vi "Rename State in Schedule.vi"(0 "Tosca in":refnum<class "Parameters.lvclass">, 5 "Old Name":string, 7 "New Name":string, 11 "error in (no error)":errorcluster) -> (4 "Tosca out":refnum<class "Parameters.lvclass">, 15 "error out":errorcluster)   [LabVIEW 2015, in "Parameters.lvclass"]
uses:
  Parameters.lvclass
  Parameters.lvclass/Parameters.ctl
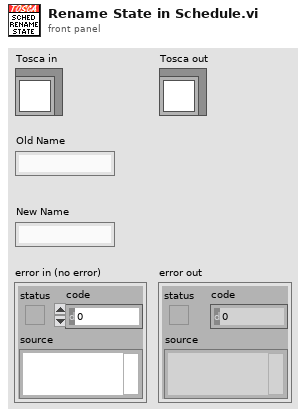
[diagram p1: front panel]
types:
  T1 = typedef "Tosca-Parameter Family.ctl" = cluster{"Name":string, "Number":i32, "Vars":T2[], "Mask":bool[][], "one each":bool}
  T2 = typedef "Tosca-Parameter Table Element.ctl" = cluster{"state":string, "chan":string, "param":string, "expr":string, "dim":T3, "value":dbl[]}
  T3 = typedef "Tosca-Parameter Dimension.ctl" = enum16{"Ind", "X", "Y"}
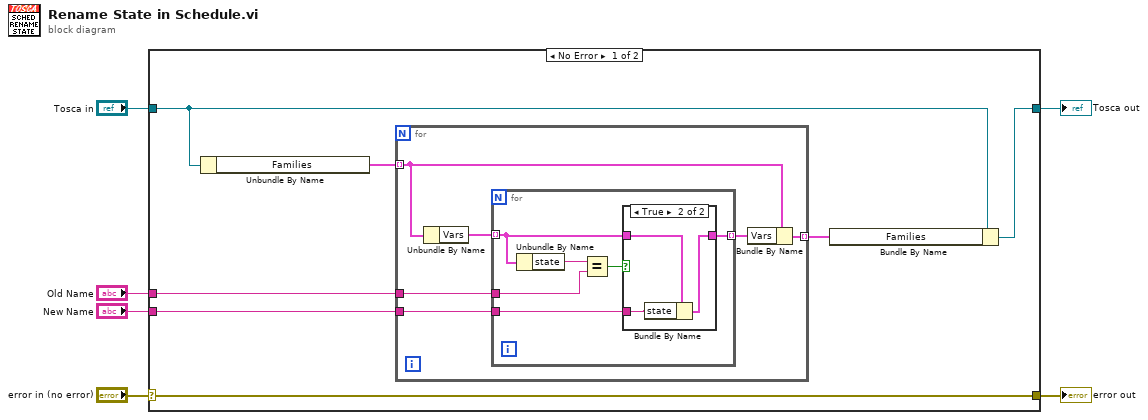
[diagram p0: block diagram]
diagram:
  n1 = case shown="No Error" "error in (no error)" {
    selector: "error in (no error)" -> [w13 w31]
    tunnel: [w13 w31] -> w5
    tunnel: [w7 w30] -> w3
    tunnel: "Tosca in" -> [w8 w30]
    tunnel: "Old Name" -> [w11 _]
    tunnel: "New Name" -> [w10 _]
    frame No Error {
      n2 = Unbundle By Name(w8) -> ("Families"=w12:T1[])
      n3 = for {
        tunnel: w12 -> [w16] mode=indexing
        tunnel: w11 -> [w18]
        tunnel: w10 -> [w17]
        tunnel: [w14] -> w9 mode=indexing
        n4 = Unbundle By Name(w16) -> ("Vars"=w19:T2[])
        n5 = for {
          tunnel: w19 -> [w22] mode=indexing
          tunnel: w18 -> [w24]
          tunnel: w17 -> [w21]
          tunnel: [w20] -> w15 mode=indexing
          n6 = Unbundle By Name(w22) -> ("state"=w25:string)
          n7 = Equal?(x=w25, y=w24) -> (x = y?=w23:bool)
          n8 = case shown="True" w23 {
            tunnel: w22 -> [w26 w29]
            tunnel: w21 -> [_ w28]
            tunnel: [w26 w27] -> w20
            frame False {
            }
            frame True {
              n9 = Bundle By Name(cluster=w29, "state"=w28) -> (w27:T2)
            }
          }
        }
        n10 = Bundle By Name(cluster=w16, "Vars"=w15) -> (w14:T1)
      }
      n11 = Bundle By Name(cluster=w8, "Families"=w9) -> (w7:refnum<class "Parameters.lvclass">)
    }
    frame Error {
    }
  }
  "error out" <- w5
  "Tosca out" <- w3
